vi "3D-SaveALLToleracnceParams.vi"(9 "Tolerance Param":string[][](table)=[["", "", ""], ["", "", ""]], 10 "名称或相对路径":string, 11 "路径":path) -> ()   [LabVIEW 2017]
uses:
  <vilib>/Utility/file.llb/Write To Spreadsheet File (string).vi
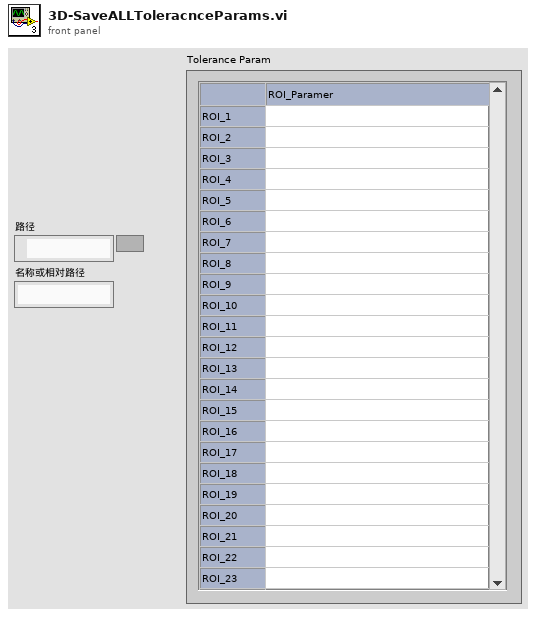
[diagram p1: front panel]
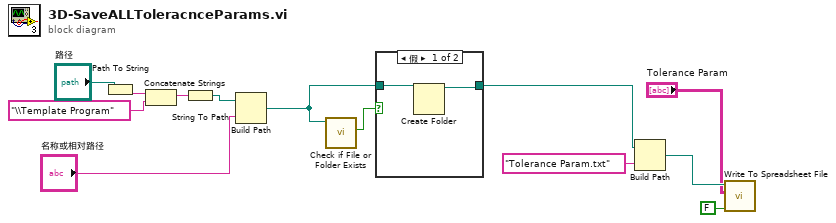
[diagram p0: block diagram]
diagram:
  n1 = Path To String(path="路径") -> (string=w13:string)
  n2 = Concatenate Strings(w13, "\\Template Program" ("字符串")) -> (w12:string)
  n3 = String To Path(string=w12) -> (path=w10:path)
  n4 = Build Path(base path=w10, name or relative path="名称或相对路径") -> (appended path=w2:path)
  n5 = call <vilib>:"Check if File or Folder Exists.vi"("path"=w2) -> ("file or folder exists?"=w3:bool)  [unwired: 8 in, 2 out]
  n6 = case shown="假" w3 {
    tunnel: w2 -> [w15 w16]
    tunnel: [w14 w16] -> w1
    frame False {
      n7 = Create Folder(path (use dialog)=w15) -> (created path=w14:path)  [unwired: 2 in, 2 out]
    }
    frame True {
    }
  }
  n8 = Build Path(base path=w1, name or relative path="Tolerance Param.txt" ("名称或相对路径")) -> (appended path=w5:path)
  n9 = call-poly <vilib>:"Write To Spreadsheet File.vi"("append to file? (new file:F)"=FALSE, "2D data"="Tolerance Param", "file path (dialog if empty)"=w5) -> ()  [unwired: 5 in, 1 out]
